vi "VNA Calset Correction - SParam.vi"(8 "error in":errorcluster, 10 "RFmxVNA Settings":T1={"Resource Name"="", "vCal Name"="", "RFmxVNA Calset Enable"=FALSE, "RFmxVNA Calset Interpolation"=FALSE, "Calset File Path"="", "RFmxVNA attenuation mode"=enum."s2p File", "RFmxVNA Port1 s2p file path"="", "RFmxVNA Port1 s-parameters orientation"=enum."Port1 Towards DUT", "RFmxVNA Port1 Power Compensation"=FALSE, "RFmxVNA Port2 s2p file path"="", "RFmxVNA Port2 s-parameters orientation"=enum."Port1 Towards DUT", "RFmxVNA Port2 Power Compensation"=FALSE, "Port1 Power Level (dBm)"=0.0, "Port1 Test Receiver Attenuation (dB)"=0.0, "Port2 Power Level (dBm)"=0.0, "Port2 Test Receiver Attenuation (dB)"=0.0, "IF Bandwidth (Hz)"=0.0, "Frequency Sweep"={"Start Frequency (Hz)"=4000000000.0, "Stop Frequency (Hz)"=26000000000.0, "Number of Points"=200}} {"Frequency Sweep"."Stop Frequency (Hz)" format="%.3p"; "Frequency Sweep"."Start Frequency (Hz)" format="%.3p"; "IF Bandwidth (Hz)" format="%.2p"; "Port2 Test Receiver Attenuation (dB)" format="%.2f"; "Port2 Power Level (dBm)" format="%.2f"; "Port1 Test Receiver Attenuation (dB)" format="%.2f"; "Port1 Power Level (dBm)" format="%.2f"}, 11 "RFmxVNA Session in":refnum<k21>) -> (0 "error out":errorcluster, 3 "RFmxVNA Session out":refnum<k21>)   [LabVIEW 2023]
uses:
  Controls/RFmxVNA Config - SParam.ctl
  <resource>/objmgr/RFmxVNA.rc
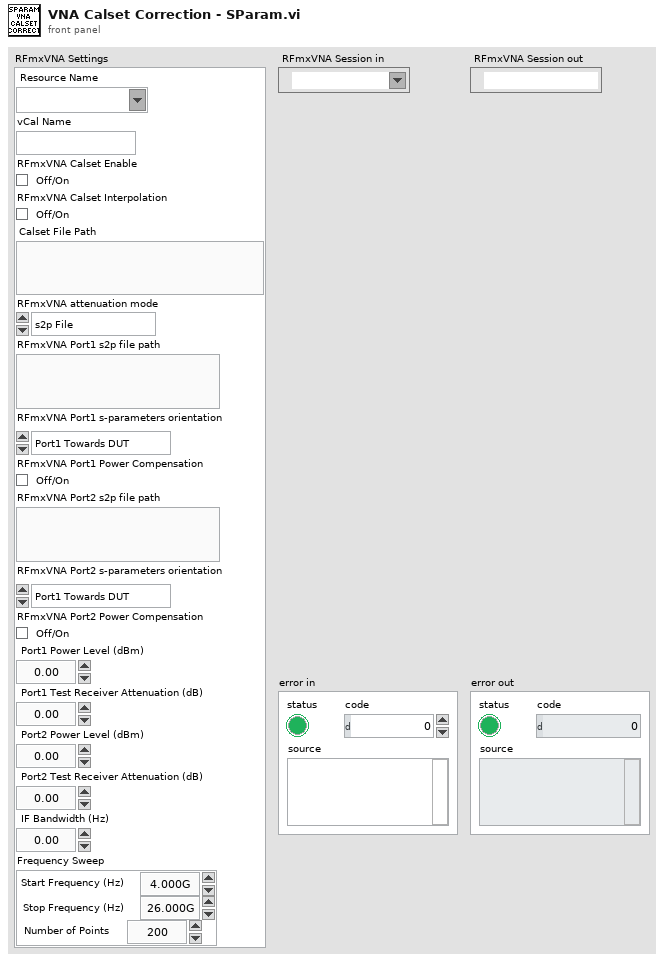
[diagram p1: front panel]
types:
  T1 = typedef "RFmxVNA Config - SParam.ctl" = cluster{"Resource Name":refnum<k15>, "vCal Name":string, "RFmxVNA Calset Enable":bool, "RFmxVNA Calset Interpolation":bool, "Calset File Path":string, "RFmxVNA attenuation mode":enum32{"<None>", "s2p File"}, "RFmxVNA Port1 s2p file path":string, "RFmxVNA Port1 s-parameters orientation":enum32{"Port1 Towards DUT", "Port2 Towards DUT"}, "RFmxVNA Port1 Power Compensation":bool, "RFmxVNA Port2 s2p file path":string, "RFmxVNA Port2 s-parameters orientation":enum32{"Port1 Towards DUT", "Port2 Towards DUT"}, "RFmxVNA Port2 Power Compensation":bool, "Port1 Power Level (dBm)":dbl, "Port1 Test Receiver Attenuation (dB)":dbl, "Port2 Power Level (dBm)":dbl, "Port2 Test Receiver Attenuation (dB)":dbl, "IF Bandwidth (Hz)":dbl, "Frequency Sweep":cluster{"Start Frequency (Hz)":dbl, "Stop Frequency (Hz)":dbl, "Number of Points":i32}}
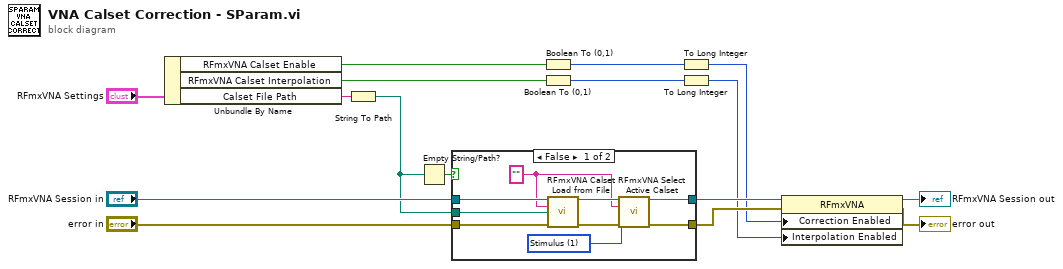
[diagram p0: block diagram]
diagram:
  n1 = Unbundle By Name("RFmxVNA Settings") -> ("RFmxVNA Calset Enable"=w8:bool, "RFmxVNA Calset Interpolation"=w7:bool, "Calset File Path"=w10:string)
  n2 = String To Path(string=w10) -> (path=w4:path)
  n3 = Empty String/Path?(string/path=w4) -> (empty?=w3:bool)
  n4 = case shown="False" w3 {
    tunnel: w4 -> [w25 _]
    tunnel: "error in" -> [w24 w26]
    tunnel: [w19 w26] -> w14
    tunnel: [w20 w27] -> w11
    tunnel: "RFmxVNA Session in" -> [w23 w27]
    frame False {
      w17 = 1 items=["None", "Stimulus"] ("Restore Configuration")
      w18 = "" ("Calset Name")
      n5 = call <vilib>:"RFmxVNA Calset Load from File.vi"("Instrument Handle In"=w23, "Calset Name"=w18, "Calset File Path"=w25, "error in (no error)"=w24) -> ("Instrument Handle Out"=w22:refnum<k21>, "error out"=w21:errorcluster)  [unwired: 10 in]
      n6 = call <vilib>:"RFmxVNA Select Active Calset.vi"("Instrument Handle In"=w22, "Calset Name"=w18, "Restore Configuration"=w17, "error in (no error)"=w21) -> ("Instrument Handle Out"=w20:refnum<k21>, "error out"=w19:errorcluster)  [unwired: 10 in]
    }
    frame True {
    }
  }
  n7 = Boolean To (0,1)(Boolean=w8) -> (0, 1=w6:i16)
  n8 = Boolean To (0,1)(Boolean=w7) -> (0, 1=w5:i16)
  n9 = To Long Integer(number=w6) -> (32bit integer=w2:i32)
  n10 = To Long Integer(number=w5) -> (32bit integer=w1:i32)
  n11 = property class="RFmxVNA"(reference=w11, error in=w14, "Correction Enabled"=w2, "Interpolation Enabled"=w1) -> (reference out=→"RFmxVNA Session out":refnum<k21>, error out=→"error out":errorcluster)
